vi "Ejercicio2_Estructura Select.vi"() -> ()   [LabVIEW 2018]
panel:
  in  "stop":bool
  in  "Tanque":dbl(slide) scale=0.0..10.0
  out "Menos de 5":bool
  out "Más de 5":bool
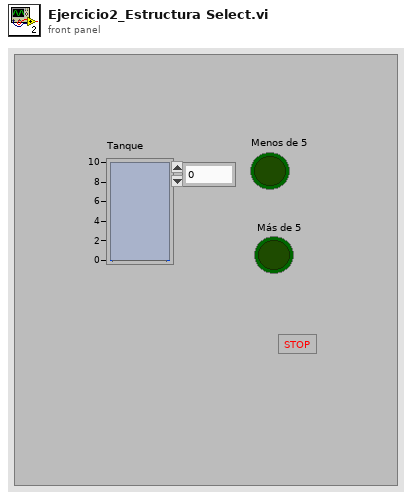
[diagram p1: front panel]
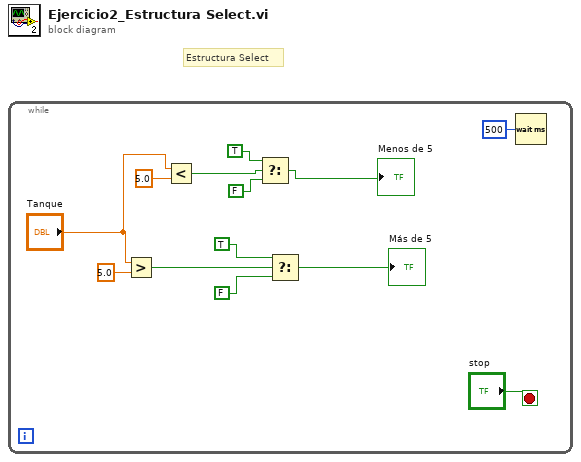
[diagram p0: block diagram]
diagram:
  # "Estructura Select"
  n1 = while {
    stop <- "stop" stop-if-true
    n2 = Greater?(x="Tanque", y=5.0) -> (0:w10:bool)
    n3 = Less?(x="Tanque", y=5.0) -> (x < y?=w4:bool)
    n4 = Select(t=TRUE, s=w4, f=FALSE) -> (s? t:f=→"Menos de 5":bool)
    n5 = Select(t=TRUE, s=w10, f=FALSE) -> (s? t:f=→"Más de 5":bool)
    n6 = Wait (ms)(milliseconds to wait=u32 500) -> ()  [unwired: 1 out]
  }
